vi "Get Controller Address.vi"(8 "error in (no error)":errorcluster, 11 "NIVS.System Definition Root In":refnum<k24>) -> (0 "error out":errorcluster, 1 "Results":T1[](array[typedef]), 2 "Names":string[](array[string]), 3 "NIVS.System Definition Root Out":refnum<k24>, 4 "Array":bool[](array[boolean]))   [LabVIEW 2016, in "ds402mgr_Helper.lvlib"]
uses:
  ds402mgr_Helper.lvlib
  NationalInstruments.VeriStand.SystemStorage
  controls/_targetDetails.ctl
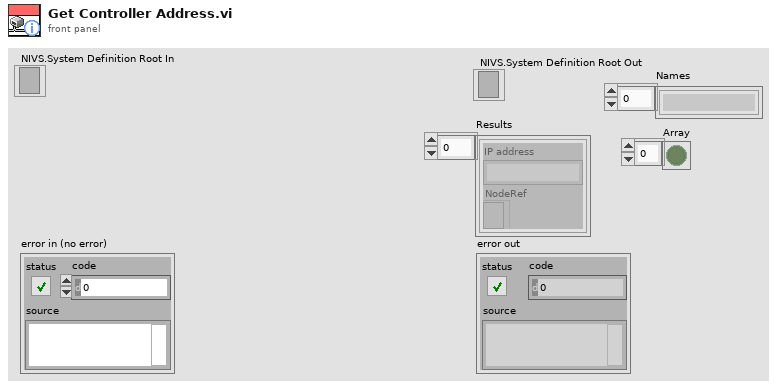
[diagram p1: front panel]
types:
  T1 = typedef "ds402mgr_Helper.lvlib/_targetDetails.ctl" = cluster{"IP address":string, "NodeRef":refnum<k24>}
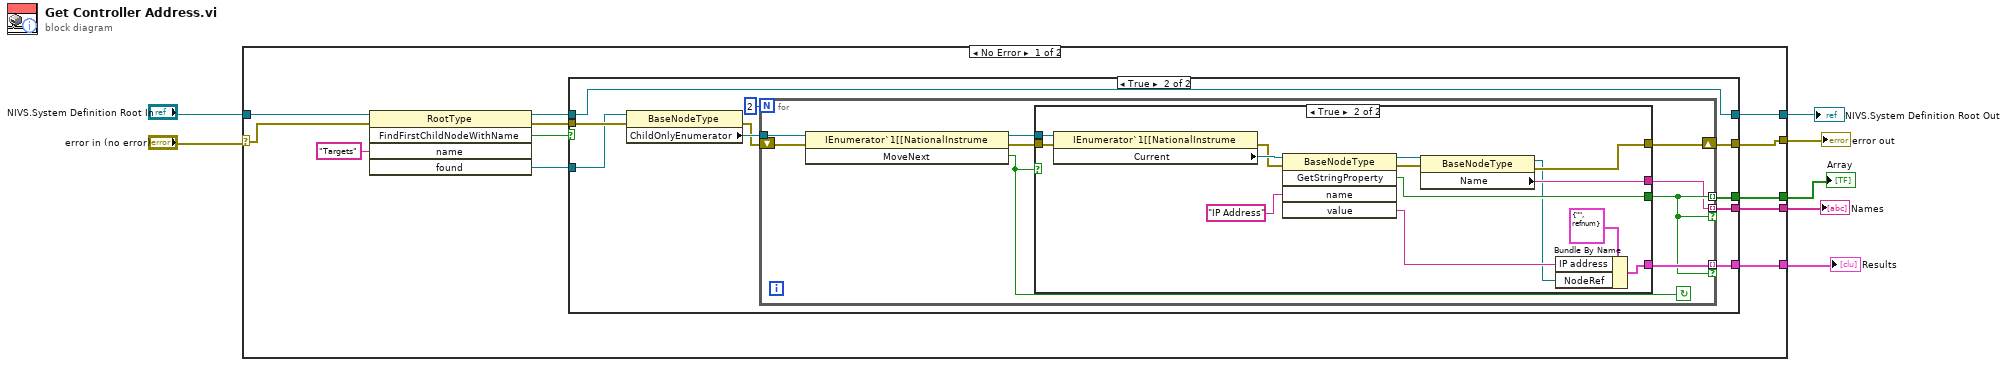
[diagram p0: block diagram]
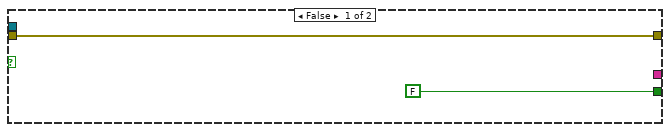
[diagram p3: hidden frame]
diagram:
  n1 = case shown="No Error" "error in (no error)" {
    selector: "error in (no error)" -> [w17 w57]
    tunnel: "NIVS.System Definition Root In" -> [w18 w58]
    tunnel: [w13 w58] -> w5
    tunnel: [w11 w57] -> w4
    tunnel: [w10 _] -> w3
    tunnel: [w9 _] -> w2
    tunnel: [w8 _] -> w1
    frame No Error {
      n2 = invoke class="RootType" method="FindFirstChildNodeWithName"(reference=w18, error in=w17, "name"="Targets") -> (reference out=w14:refnum<k24>, error out=w15:errorcluster, "FindFirstChildNodeWithName"=w16:bool, "found"=w12:refnum<k24>)  [unwired: 2 in, 1 out]
      n3 = case shown="True" w16 {
        tunnel: w15 -> [w20 w31]
        tunnel: w14 -> [w21 w30]
        tunnel: [w21 w30] -> w13
        tunnel: w12 -> [_ w29]
        tunnel: [w20 w24] -> w11
        tunnel: [_ w25] -> w10
        tunnel: [_ w23] -> w9
        tunnel: [_ w22] -> w8
        frame False {
        }
        frame True {
          n4 = property class="BaseNodeType"(reference=w29, error in=w31) -> (error out=w27:errorcluster, "ChildOnlyEnumerator"=w28:refnum<k24>)  [unwired: 1 out]
          n5 = for {
            N: 2 -> [_]
            tunnel: w28 -> [w40]
            tunnel: [w32] -> w22 mode=indexing if=w33
            tunnel: [w33] -> w25 mode=indexing
            shift-right: [w35] -> w24
            shift-left: w27 -> [w39]
            tunnel: [w34] -> w23 mode=indexing if=w33
            stop <- w36 continue-if-true
            n6 = invoke class="IEnumerator`1[[NationalInstrume" method="MoveNext"(reference=w40, error in=w39) -> (reference out=w38:refnum<k24>, error out=w37:errorcluster, "MoveNext"=w36:bool)  [unwired: 1 in]
            n7 = case shown="True" w36 {
              tunnel: [FALSE ("GetStringProperty") w53] -> w33
              tunnel: w38 -> [_ w52]
              tunnel: w37 -> [w41 w51]
              tunnel: [w41 w45] -> w35
              tunnel: [_ w49] -> w34
              tunnel: [_ w44] -> w32
              frame False {
              }
              frame True {
                n8 = property class="IEnumerator`1[[NationalInstrume"(reference=w52, error in=w51) -> (error out=w55:errorcluster, "Current"=w56:refnum<k24>)  [unwired: 1 out]
                n9 = invoke class="BaseNodeType" method="GetStringProperty"(reference=w56, error in=w55, "name"="IP Address") -> (reference out=w47:refnum<k24>, error out=w46:errorcluster, "GetStringProperty"=w53:bool, "value"=w48:string)  [unwired: 2 in, 1 out]
                n10 = property class="BaseNodeType"(reference=w47, error in=w46) -> (reference out=w43:refnum<k24>, error out=w45:errorcluster, "Name"=w44:string)
                n11 = Bundle By Name(cluster=T1 {"IP address"="", "NodeRef"=refnum} ("Results"), "IP address"=w48, "NodeRef"=w43) -> (w49:T1)
              }
            }
          }
        }
      }
    }
    frame Error {
    }
  }
  "NIVS.System Definition Root Out" <- w5
  "error out" <- w4
  "Results" <- w2
  "Names" <- w1
  "Array" <- w3
